vi "ApplySelectedLayout.vi"(8 "error in (no error)":errorcluster, 9 "Layout index":i32, 10 "Col array":refnum<class "Column.lvclass">[](array[class]), 11 "Tbl Refnum":refnum<vi>) -> (0 "error out":errorcluster)   [LabVIEW 2013]
doc: "Push column width changes to Setlist Table. If the width of data columns shown is less than the content rectangle, adjust the view so that the full table width is showing data.\nThis VI is read-only w.r.t column data."
uses:
  ColumnVIs/Column/Column.lvclass
  <vilib>/Utility/miscctls.llb/LVRowAndColumnUnsignedTypeDef.ctl
  <vilib>/Utility/miscctls.llb/LVBoundsTypeDef.ctl
  <vilib>/Utility/miscctls.llb/LVRowAndColumnTypeDef.ctl
panel:
  out "move scrollbar?":bool
  out "Content Rect Bounds":T1
  out "Index Values":T2
  out "total width":u32
  out "Set Width Array":u32[](array[numeric])
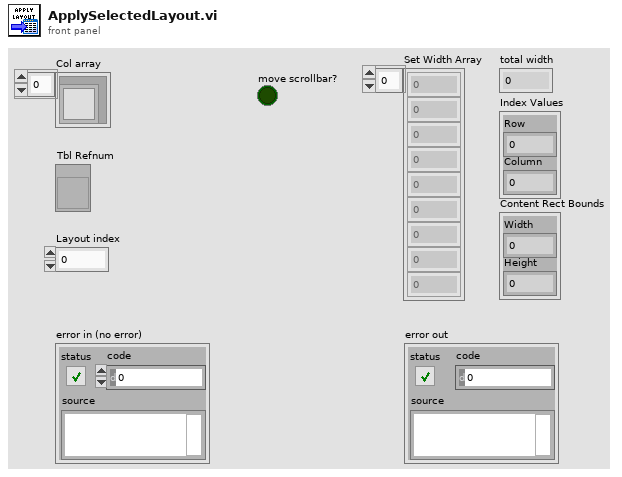
[diagram p1: front panel]
types:
  T1 = typedef "LVBoundsTypeDef.ctl" = cluster{"Width":u32, "Height":u32}
  T2 = typedef "LVRowAndColumnUnsignedTypeDef.ctl" = cluster{"Row":u32, "Column":u32}
  T3 = typedef "LVRowAndColumnTypeDef.ctl" = cluster{"Row":i32, "Column":i32}
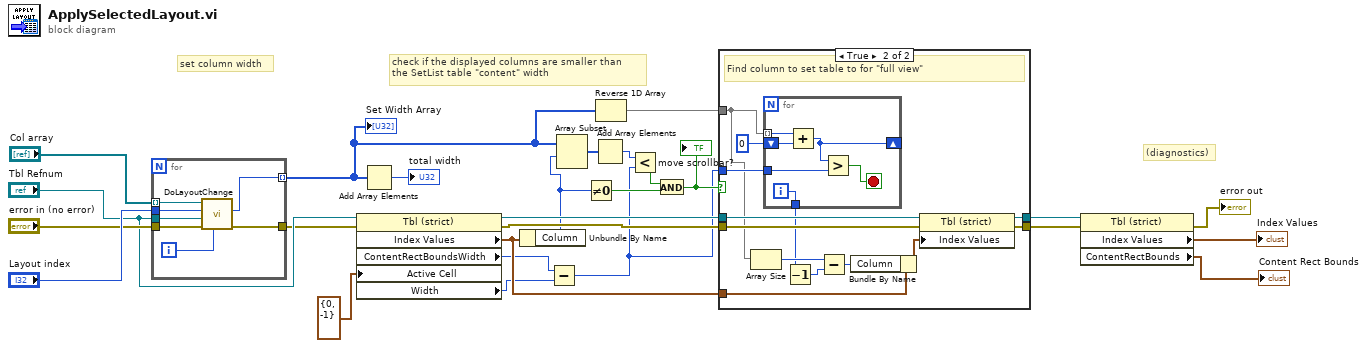
[diagram p0: block diagram]
diagram:
  # "check if the displayed columns are smaller than \nthe SetList table \"content\" width"
  # "set column width"
  # "(diagnostics)"
  n1 = for {
    tunnel: "Tbl Refnum" -> [w31]
    tunnel: "error in (no error)" -> [w32]
    tunnel: "Col array" -> [w33] mode=indexing
    tunnel: [w29] -> w18
    tunnel: "Layout index" -> [w28]
    tunnel: [w27] -> w6 mode=indexing
    i -> [w30]
    n2 = call "DoLayoutChange.vi"("Column"=w30, "error in (no error)"=w32, "Tbl Refnum"=w31, "Layout index"=w28, "Column in"=w33) -> ("error out"=w29:errorcluster, "Set Width"=w27:u32)  [unwired: 4 in, 1 out]
  }
  "Set Width Array" <- w6
  n3 = property class="Tbl (strict)"(reference="Tbl Refnum", error in=w18, "Active Cell"=T3 {"Row"=0, "Column"=-1} ("Active Cell:Active Cell")) -> (reference out=w15:refnum<vi>, error out=w14:errorcluster, "Index Values"=w11:T2, "ContentRectBoundsWidth"=w3:i32, "Width"=w1:u32)
  n4 = Add Array Elements(numeric array=w6) -> (sum=→"total width":u32)
  n5 = Unbundle By Name(w11) -> ("Column"=w10:u32)
  n6 = Subtract(x=w3, y=w1) -> (x-y=w2:u32)
  n7 = Array Subset(array=w6, index=w10) -> (w17:u32[])  [unwired: 1 in]
  n8 = Not Equal To 0?(x=w10) -> (x != 0?=w8:bool)
  n9 = Add Array Elements(numeric array=w17) -> (sum=w16:u32)
  n10 = Reverse 1D Array(array=w6) -> (reversed array=w5:u32[])
  n11 = Less?(x=w16, y=w2) -> (x < y?=w9:bool)
  n12 = And(x=w9, y=w8) -> (x .and. y?=w7:bool)
  "move scrollbar?" <- w7
  n13 = case shown="True" w7 {
    tunnel: w15 -> [w35 w48]
    tunnel: w14 -> [w34 w47]
    tunnel: [w35 w46] -> w13
    tunnel: [w34 w45] -> w12
    tunnel: w11 -> [_ w44]
    tunnel: w5 -> [_ w40]
    tunnel: w2 -> [_ w41]
    frame False {
      # "Columns already take up full view: do nothing"
    }
    frame True {
      # "Find column to set table to for \"full view\""
      n14 = Array Size(array=w40) -> (size(s)=w39:i32)
      n15 = for {
        tunnel: w40 -> [w54] mode=indexing
        shift-right: [w51] -> _
        shift-left: u32 0 ("y") -> [w53]
        tunnel: w41 -> [w50]
        tunnel: [w49] -> w37
        i -> [w49]
        stop <- w52 stop-if-true
        n16 = Add(x=w54, y=w53) -> (x+y=w51:u32)
        n17 = Greater?(x=w51, y=w50) -> (0:w52:bool)
      }
      n18 = Decrement(x=w37) -> (x-1=w36:i32)
      n19 = Subtract(x=w39, y=w36) -> (x-y=w38:i32)
      n20 = Bundle By Name(cluster=w44, "Column"=w38) -> (w43:T2)
      n21 = property class="Tbl (strict)"(reference=w48, error in=w47, "Index Values"=w43) -> (reference out=w46:refnum<vi>, error out=w45:errorcluster)
    }
  }
  n22 = property class="Tbl (strict)"(reference=w13, error in=w12) -> (error out=→"error out":errorcluster, "Index Values"=→"Index Values":T2, "ContentRectBounds"=→"Content Rect Bounds":T1)  [unwired: 1 out]
